vi "XY Graph Get Tool Panels Visibility.vi"(8 "error in (no error)":errorcluster, 11 "XYGraph in":T1) -> (0 "error out":errorcluster, 1 "Was Tag Found?":bool, 2 "Graph Tool Panels Visibility":T2, 3 "XYGraph out":T1)   [LabVIEW 2021, in "XY Graph Add-Ons.lvlib"]
uses:
  XY Graph Add-Ons.lvlib
  XY Graph Tool Panels Visibility.ctl
  XY Graph Refnum.ctl
  XY Graph Property Tag List.ctl
  <vilib>/UserTags/UserTags.lvlib
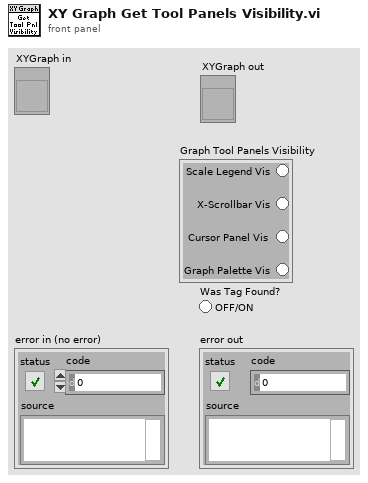
[diagram p1: front panel]
types:
  T1 = typedef "XY Graph Add-Ons.lvlib/XY Graph Refnum.ctl" = refnum<vi>
  T2 = typedef "XY Graph Add-Ons.lvlib/XY Graph Tool Panels Visibility.ctl" = cluster{"Scale Legend Vis":bool, "X-Scrollbar Vis":bool, "Cursor Panel Vis":bool, "Graph Palette Vis":bool}
  T3 = typedef "XY Graph Add-Ons.lvlib/XY Graph Property Tag List.ctl" = enum16{"Max Legend Size", "Preserved Plots", "XScales.GridColors", "YScales.GridColors", "TipStrip String", "TipStrip Visible", "Tool Panels Visibility", "Plots Metadata"}
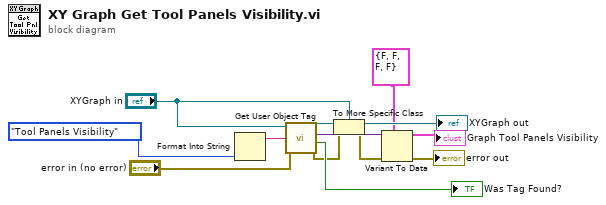
[diagram p0: block diagram]
diagram:
  n1 = Format Into String(XY_Graph_Property_Tag_List."Tool Panels Visibility" ("XY Graph Property Tag")) -> (resulting string=w12:string)  [unwired: 3 in, 1 out]
  n2 = call <vilib>:"Get User Object Tag.vi"("error in (no error)"="error in (no error)", "Tag Name"=w12, "Generic Refnum"="XYGraph in") -> ("error out"=w4:errorcluster, "Was Tag Found?"=→"Was Tag Found?":bool, "Value"=w9:variant, "dup Generic Refnum"=w7:refnum<vi>)  [unwired: 5 in]
  n3 = To More Specific Class(target class="XYGraph in", reference=w7, error in=w4) -> (specific class reference=→"XYGraph out":T1, error out=w3:errorcluster)
  n4 = Variant To Data(error in=w3, type=T2 {"Scale Legend Vis"=FALSE, "X-Scrollbar Vis"=FALSE, "Cursor Panel Vis"=FALSE, "Graph Palette Vis"=FALSE} ("Graph Tool Panels Visibility"), Variant=w9) -> (data=→"Graph Tool Panels Visibility":T2, error out=→"error out":errorcluster)
